vi "Read Group Info.vi"(10 "Neuron Type":T1, 11 "Grid in":refnum<class "Grid.lvclass">) -> (1 "Index":i32, 2 "N":i32, 3 "Grid out":refnum<class "Grid.lvclass">)   [LabVIEW 2013, in "Grid.lvclass"]
doc: "This method returns the information of an specific type of Neurons and the IDs of the neurons belonging to that type(group)"
uses:
  Grid.lvclass
  Controls/Type of Neuron.ctl
  Grid.lvclass/Grid.ctl
  Neuron/Neuron.lvclass/Neuron.ctl
  Neuron/Neuron.lvclass
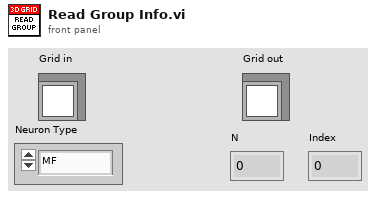
[diagram p1: front panel]
types:
  T1 = typedef "Type of Neuron.ctl" = enum16{"MF", "BA", "GO", "GC", "PC", "LU", "Glia (Dummy)"}
  T2 = typedef "Neuron Info.ctl" = cluster{"N":i32, "Radius":dbl, "Type":T1, "Color":u32}[]
  T3 = cluster{"N":i32, "Radius":dbl, "Type":T1, "Color":u32}
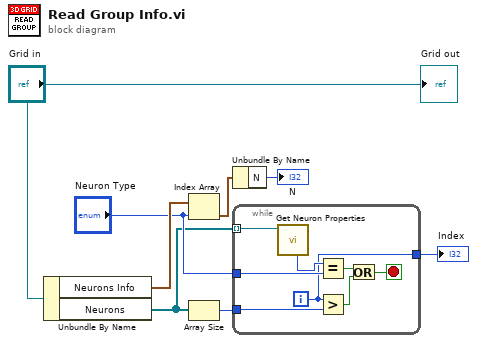
[diagram p0: block diagram]
diagram:
  n1 = Unbundle By Name("Grid in") -> ("Neurons Info"=w7:T2, "Neurons"=w2:refnum<class "Neuron.lvclass">[])
  n2 = Index Array(array=w7, index="Neuron Type") -> (element=w6:T3)
  n3 = Array Size(array=w2) -> (size(s)=w1:i32)
  n4 = Unbundle By Name(w6) -> ("N"=→"N":i32)
  n5 = while {
    tunnel: w2 -> [w16] mode=indexing
    tunnel: "Neuron Type" -> [w14]
    tunnel: [w12] -> w3
    tunnel: w1 -> [w11]
    i -> [w12]
    stop <- w10 stop-if-true
    n6 = call "Get Neuron Properties.vi"("Neuron in"=w16) -> ("Group"=w15:T1)  [unwired: 5 in, 5 out]
    n7 = Equal?(x=w15, y=w14) -> (x = y?=w13:bool)
    n8 = Greater?(x=w12, y=w11) -> (0:w9:bool)
    n9 = Or(x=w13, y=w9) -> (x .or. y?=w10:bool)
  }
  "Index" <- w3
  "Grid out" <- "Grid in"
